vi "Create New Container.vi"(11 "Sequence Context":refnum<k7>) -> (0 "error out":errorcluster)   [LabVIEW 2011]
doc: "This VI creates a new complex PropertyObject container as a Local variable and the fields are added using the NewSubProperty methods."
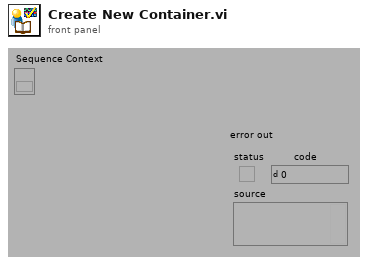
[diagram p1: front panel]
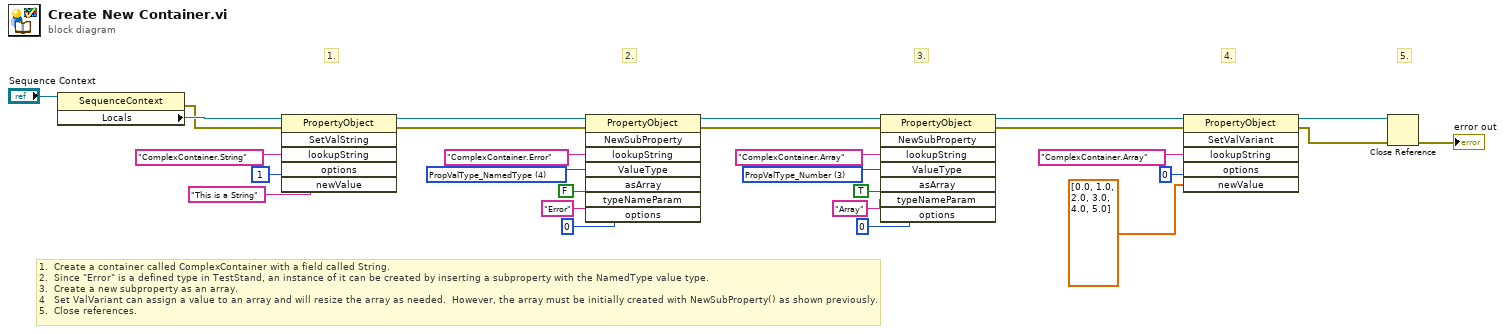
[diagram p0: block diagram]
diagram:
  w12 = 3 items=["PropValType_Container", "PropValType_String", "PropValType_Boolean", "PropValType_Number", "PropValType_NamedType", "PropValType_Reference", "PropValType_Array"] ("ValueType")
  w19 = 4 items=["PropValType_Container", "PropValType_String", "PropValType_Boolean", "PropValType_Number", "PropValType_NamedType", "PropValType_Reference", "PropValType_Array"] ("ValueType")
  # "5."
  # "4."
  # "3."
  # "2."
  # "1."
  # "1.  Create a container called ComplexContainer with a field called String.\n2.  Since \"Error\" is a defined type in TestStand, an instance of it can be created by inserting a subproperty with the NamedType value type.\n3.  Create a new subproperty as an array.\n4   Set ValVariant can assign a value to an array and will resize the array as needed.  However, the array must be initially created with NewSubProperty() as shown previously.\n5.  Close references."
  n1 = property class="SequenceContext"(reference="Sequence Context") -> (error out=w26:errorcluster, "Locals"=w27:refnum<k7>)  [unwired: 1 in, 1 out]
  n2 = invoke class="PropertyObject" method="SetValString"(reference=w27, error in=w26, "lookupString"="ComplexContainer.String", "options"=1, "newValue"="This is a String") -> (reference out=w22:refnum<k7>, error out=w21:errorcluster)  [unwired: 1 in, 4 out]
  n3 = invoke class="PropertyObject" method="NewSubProperty"(reference=w22, error in=w21, "lookupString"="ComplexContainer.Error", "ValueType"=w19, "asArray"=FALSE, "typeNameParam"="Error", "options"=0) -> (reference out=w15:refnum<k7>, error out=w14:errorcluster)  [unwired: 1 in, 6 out]
  n4 = invoke class="PropertyObject" method="NewSubProperty"(reference=w15, error in=w14, "lookupString"="ComplexContainer.Array", "ValueType"=w12, "asArray"=TRUE, "typeNameParam"="Array", "options"=0) -> (reference out=w2:refnum<k7>, error out=w3:errorcluster)  [unwired: 1 in, 6 out]
  n5 = invoke class="PropertyObject" method="SetValVariant"(reference=w2, error in=w3, "lookupString"="ComplexContainer.Array", "options"=0, "newValue"=dbl[] [0.0, 1.0, 2.0, 3.0, 4.0, 5.0]) -> (reference out=w5:refnum<k7>, error out=w1:errorcluster)  [unwired: 1 in, 4 out]
  n6 = Close Reference(reference=w5, error in (no error)=w1) -> (error out=→"error out":errorcluster)
